vi "NI VeriStand - Start Data Logging.vi"(8 "error in (no error)":errorcluster, 9 "Data Log File Configuration":T1={"File Path"=path "", "Description"="", "Trigger"={"Type"=enum."None", "Channel Path"="", "High Limit"=0.0, "Low Limit"=0.0}, "Replace File"=FALSE, "Rate [Hz]"=1.0, "File Properties"=[], "Channels"=[]}, 10 "Data Log Configuration Name":string, 11 "WorkspaceManager in":T6) -> (0 "error out":errorcluster, 3 "WorkspaceManager out":T6)   [LabVIEW 2020, in "NI_VS Workspace ExecutionAPI.lvlib"]
doc: "Starts logging data for the specified <B>Data Log Configuration Name</B>."
uses:
  <vilib>/NI VeriStand/Execution/Workspace/NI_VS Workspace ExecutionAPI.lvlib
  <vilib>/NI VeriStand/Execution/Workspace/WorkspaceAPI.ctl
  NationalInstruments.VeriStand.ClientAPI
  <vilib>/NI VeriStand/Execution/Workspace/LogFileConfiguration.ctl
  <vilib>/NI VeriStand/Execution/Workspace/LogFileTriggerConfiguration.ctl
  <vilib>/NI VeriStand/Execution/Workspace/LogFileTriggerType.ctl
  <vilib>/NI VeriStand/Execution/Workspace/LogProperty.ctl
  <vilib>/NI VeriStand/Execution/Workspace/LogChannelConfiguration.ctl
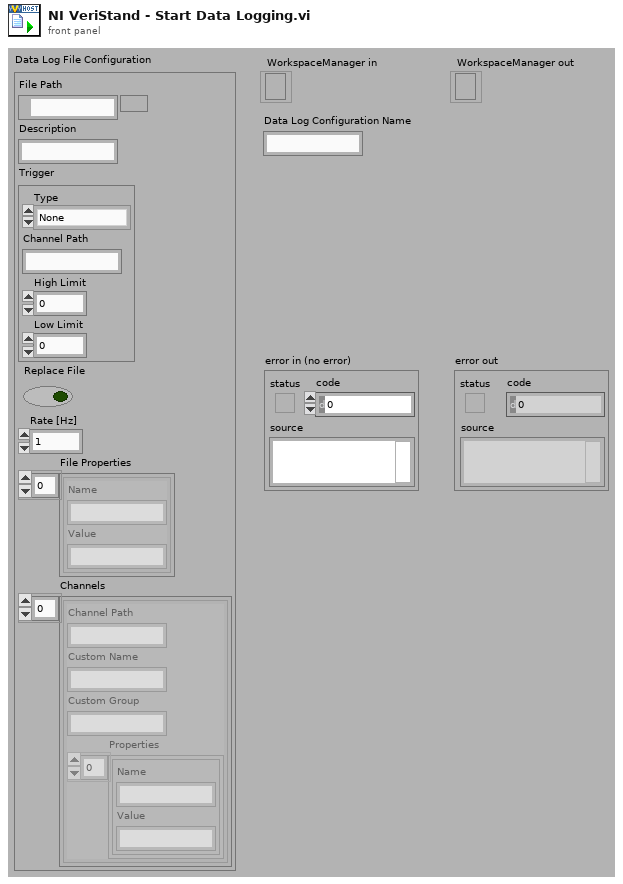
[diagram p1: front panel]
types:
  T1 = typedef "NI_VS Workspace ExecutionAPI.lvlib/LogFileConfiguration.ctl" = cluster{"File Path":path, "Description":string, "Trigger":T2, "Replace File":bool, "Rate [Hz]":dbl, "File Properties":T4[], "Channels":T5[]}
  T2 = typedef "NI_VS Workspace ExecutionAPI.lvlib/LogFileTriggerConfiguration.ctl" = cluster{"Type":T3, "Channel Path":string, "High Limit":dbl, "Low Limit":dbl}
  T3 = typedef "NI_VS Workspace ExecutionAPI.lvlib/LogFileTriggerType.ctl" = enum16{"None", "In Limits", "Out of Limits"}
  T4 = typedef "NI_VS Workspace ExecutionAPI.lvlib/LogProperty.ctl" = cluster{"Name":string, "Value":string}
  T5 = typedef "NI_VS Workspace ExecutionAPI.lvlib/LogChannelConfiguration.ctl" = cluster{"Channel Path":string, "Custom Name":string, "Custom Group":string, "Properties":T4[]}
  T6 = typedef "NI_VS Workspace ExecutionAPI.lvlib/WorkspaceAPI.ctl" = refnum<k24>
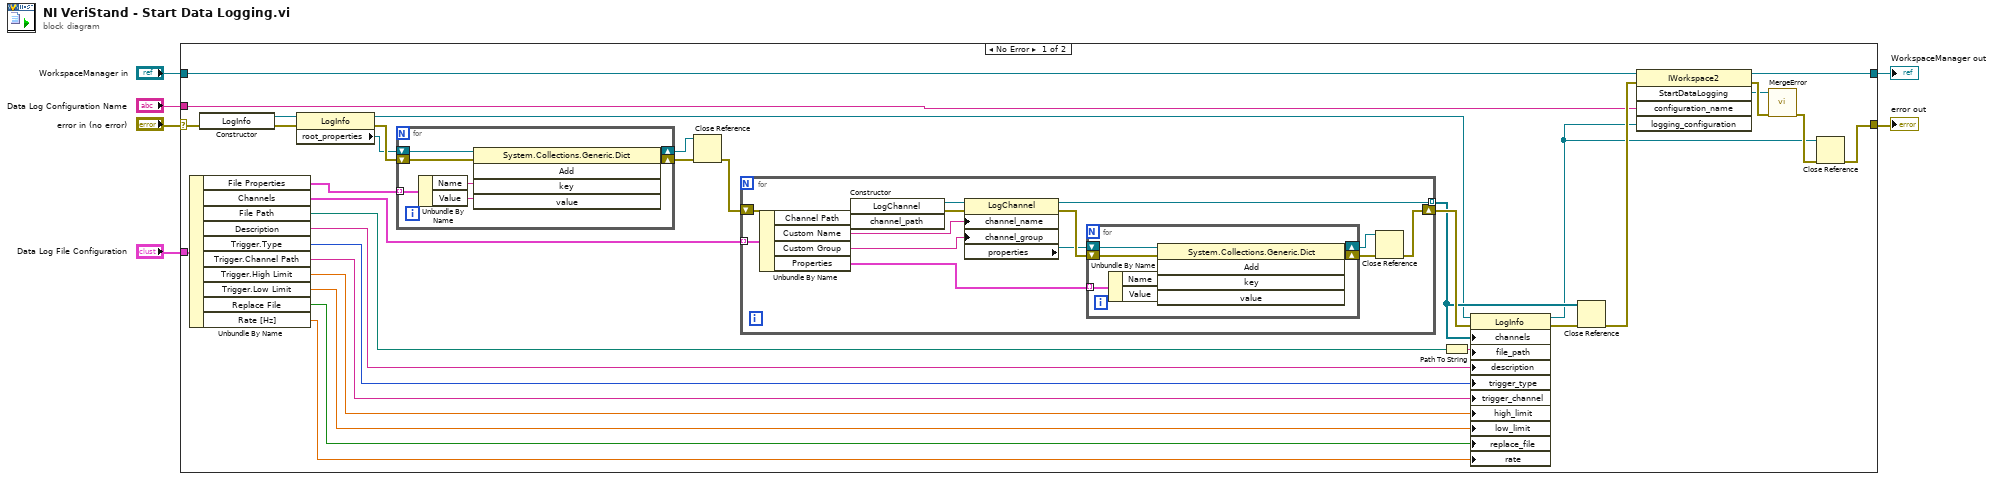
[diagram p0: block diagram]
diagram:
  n1 = case shown="No Error" "error in (no error)" {
    selector: "error in (no error)" -> [w13 w68]
    tunnel: "WorkspaceManager in" -> [w29 w69]
    tunnel: [w28 w69] -> w5
    tunnel: "Data Log Configuration Name" -> [w27 _]
    tunnel: "Data Log File Configuration" -> [w26 _]
    tunnel: [w7 w68] -> w2
    frame No Error {
      n2 = Unbundle By Name(w26) -> ("File Properties"=w25:T4[], "Channels"=w24:T5[], "File Path"=w21:path, "Description"=w20:string, "Trigger.Type"=w19:T3, "Trigger.Channel Path"=w18:string, "Trigger.High Limit"=w17:dbl, "Trigger.Low Limit"=w16:dbl, "Replace File"=w15:bool, "Rate [Hz]"=w14:dbl)
      n3 = constructor class="LogInfo"(error in=w13) -> (reference out=w34:refnum<k24>, error out=w33:errorcluster)  [unwired: 2 in, 1 out]
      n4 = property class="LogInfo"(reference=w34, error in=w33) -> (reference out=w10:refnum<k24>, error out=w36:errorcluster, "root_properties"=w32:refnum<k24>)
      n5 = for {
        shift-right: [w43] -> w30
        shift-left: w32 -> [w45]
        shift-right: [w44] -> w31
        shift-left: w36 -> [w46]
        tunnel: w25 -> [w42] mode=indexing
        n6 = Unbundle By Name(w42) -> ("Name"=w41:string, "Value"=w40:string)
        n7 = invoke class="System.Collections.Generic.Dict" method="Add"(reference=w45, error in=w46, "key"=w41, "value"=w40) -> (reference out=w43:refnum<k24>, error out=w44:errorcluster)  [unwired: 1 in, 3 out]
      }
      n8 = Close Reference(reference=w30, error in (no error)=w31) -> (error out=w23:errorcluster)
      n9 = for {
        tunnel: [w51] -> w11 mode=indexing
        tunnel: w24 -> [w59] mode=indexing
        shift-right: [w49] -> w37
        shift-left: w23 -> [w48]
        n10 = Unbundle By Name(w59) -> ("Channel Path"=w58:string, "Custom Name"=w55:string, "Custom Group"=w54:string, "Properties"=w47:T4[])
        n11 = constructor class="LogChannel"(error in=w48, "channel_path"=w58) -> (reference out=w57:refnum<k24>, error out=w56:errorcluster)  [unwired: 2 in, 2 out]
        n12 = property class="LogChannel"(reference=w57, error in=w56, "channel_name"=w55, "channel_group"=w54) -> (reference out=w51:refnum<k24>, error out=w60:errorcluster, "properties"=w53:refnum<k24>)
        n13 = for {
          shift-right: [w66] -> w52
          shift-left: w53 -> [w67]
          shift-right: [w64] -> w50
          shift-left: w60 -> [w65]
          tunnel: w47 -> [w63] mode=indexing
          n14 = Unbundle By Name(w63) -> ("Name"=w62:string, "Value"=w61:string)
          n15 = invoke class="System.Collections.Generic.Dict" method="Add"(reference=w67, error in=w65, "key"=w62, "value"=w61) -> (reference out=w66:refnum<k24>, error out=w64:errorcluster)  [unwired: 1 in, 3 out]
        }
        n16 = Close Reference(reference=w52, error in (no error)=w50) -> (error out=w49:errorcluster)
      }
      n17 = Path To String(path=w21) -> (string=w35:string)
      n18 = property class="LogInfo"(reference=w10, error in=w37, "channels"=w11, "file_path"=w35, "description"=w20, "trigger_type"=w19, "trigger_channel"=w18, "high_limit"=w17, "low_limit"=w16, "replace_file"=w15, "rate"=w14) -> (reference out=w8:refnum<k24>, error out=w12:errorcluster)
      n19 = Close Reference(reference=w11, error in (no error)=w12) -> (error out=w39:errorcluster)
      n20 = invoke class="IWorkspace2" method="StartDataLogging"(reference=w29, error in=w39, "configuration_name"=w27, "logging_configuration"=w8) -> (reference out=w28:T6, error out=w38:errorcluster, "StartDataLogging"=w22:refnum<k24>)  [unwired: 1 in, 2 out]
      n21 = call <vilib>:"MergeError.vi"("error in (no error)"=w38, "Error"=w22) -> ("error out"=w9:errorcluster)  [unwired: 9 out]
      n22 = Close Reference(reference=w8, error in (no error)=w9) -> (error out=w7:errorcluster)
    }
    frame Error {
    }
  }
  "WorkspaceManager out" <- w5
  "error out" <- w2
